vi "MasterAquisitionFile_FP_NoStim.vi"() -> ()   [LabVIEW 2020]
uses:
  <vilib>/vision/driver/IMAQdx.llb/IMAQdx Camera Control Mode.ctl
  <vilib>/vision/driver/IMAQdx.llb/IMAQdx Acquisition Mode.ctl
  <vilib>/userDefined/High Color/IMAQdx.ctl
  <vilib>/vision/driver/IMAQdx.llb/IMAQdx Buffer Number Mode.ctl
  <vilib>/DAQmx/read.llb/DAQmx Read (Digital 1D Bool 1Chan 1Samp).vi
  <vilib>/DAQmx/read.llb/DAQmx Read (Analog 1D Wfm NChan NSamp).vi
  <vilib>/DAQmx/create/channels.llb/DAQmx Create Channel (DI-Digital Input).vi
  <vilib>/DAQmx/miscellaneous.llb/DAQmx Fill In Error Info.vi
  <vilib>/DAQmx/create/channels.llb/DAQmx Create Channel (AI-Voltage-Basic).vi
  <vilib>/DAQmx/configure/timing.llb/DAQmx Timing (Sample Clock).vi
  <vilib>/DAQmx/configure/trigger.llb/DAQmx Start Trigger (Digital Edge).vi
  <vilib>/DAQmx/create/channels.llb/DAQmx Create Channel (CO-Pulse Generation-Frequency).vi
  <vilib>/DAQmx/configure/timing.llb/DAQmx Timing (Implicit).vi
  <vilib>/vision/driver/NI_Vision_Acquisition_Software.lvlib
  <resource>/objmgr/imaqdx.rc
panel:
  out "?":bool[](array[boolean])=[TRUE]
  out "Hexadecimal Data":u32=1 format="%x"
  out "Doric Trig":bool
  in  "Analog Input Channels":tag="Dev1/ai3:4, Dev1/ai7:13"
  out "?":T1(plugin-control)
  in  "stop":bool
  out "?":T1(plugin-control)
  out "Behavior Cam Fs":dbl(knob) scale=0.0..200.0
  out "Behav Cam":bool
  out "Whisk Cam":bool
  out "Analog Data":bool
  out "Time Elapsed (Min)":cluster{dbl, dbl}(slide)={16.0, 0.0} scale=0.0..16.0 scale format="%#_2g"
  out "Saving":bool
  out "Analog Samples":i32
  in  "Device Analog Channel Labels":string[](array[string])=["AudSol", "560LH", "forceSensor", "hipp", "cortRH", "cortLH", "EMG", "LPadSol", "RPadSol"]
  in  "?":cluster{"Analog Fs":u16}={"Analog Fs"=20000} {"Analog Fs" format="%0.0f"}
  in  "?":cluster{"WhiskerCam Fs":u16}={"WhiskerCam Fs"=150}
  out "Notes Size":i32=7
  out "Notes Reversed":string[](array[string])=["Experimenter", "Animal ID", "Isoflurane time", "Amplifier Gain", "Session ID", "Hemisphere", "Solenoid PSI"]
  out "Notes Array":string[](array[string])=["Solenoid PSI", "Hemisphere", "Session ID", "Amplifier Gain", "Isoflurane time", "Animal ID", "Experimenter"]
  in  "Notes:":T2={"Experimenter"="Kevin\n", "Animal ID"="T235", "Isoflurane time"="1250", "Amplifier Gain"="10000", "Session ID"="Imaging Session One", "Hemisphere"="RH", "Solenoid PSI"="10"}
  in  "Target Path":path=path "C:/Users/klt8/Documents/T236" caption="Final Saved File Location"
  out "Dropped":u32(slide) caption="WhiskerCam" scale=0.0..150.0
  out "Current File Name":string="210916_14_47_27"
  in  "Time (min)":dbl(knob)=15.5 min=0.5 max=20.0 step=0.5 scale=0.0..20.0 scale format="%#_3g"
  in  "Temp Path":path=path "C:/Users/klt8/Documents/LabVIEW Temp Data" caption="Temporary File Path"
  out "Last Whisk Buffer":u32
  out "Whisker Cam Fs":dbl(knob) scale=0.0..200.0 scale format="%#1_6g"
  # "Notes"
  # "Dropped Frames"
  # "Analog Fs"
  # "Whisker Fs"
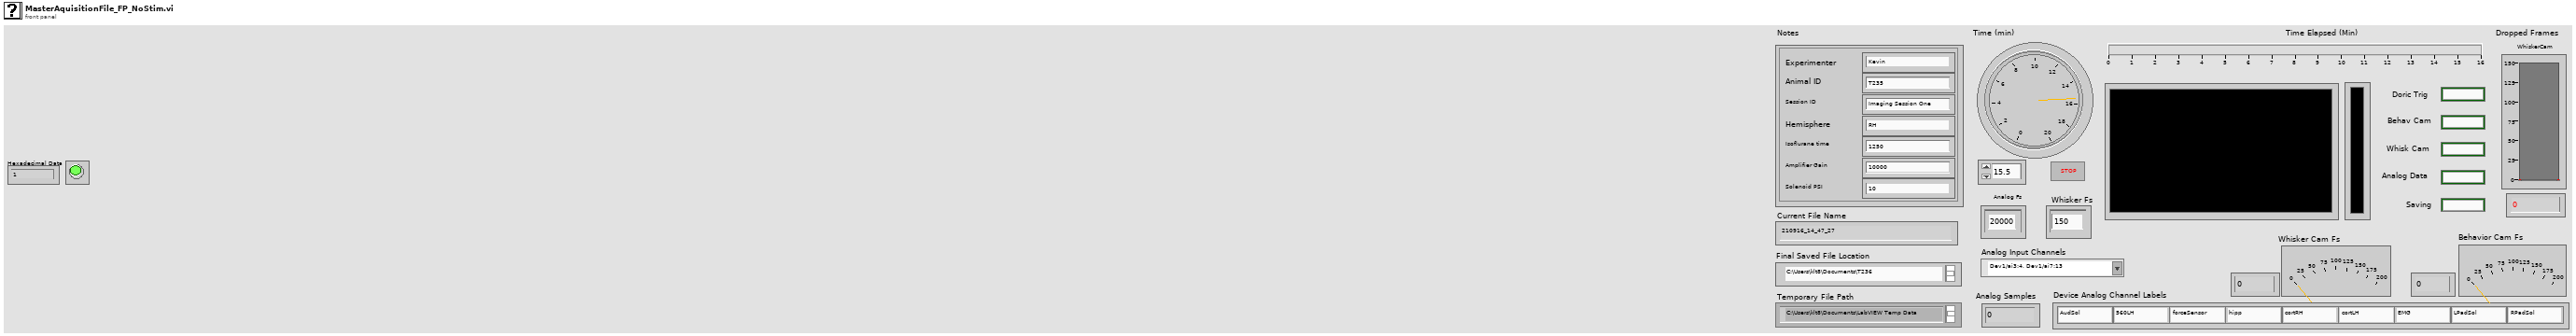
[diagram p1: front panel]
types:
  T1 = typedef "IMAQ Image.ctl" = refnum<image>
  T2 = cluster{"Experimenter":string, "Animal ID":string, "Isoflurane time":string, "Amplifier Gain":string, "Session ID":string, "Hemisphere":string, "Solenoid PSI":string}
  T3 = typedef "IMAQdx.ctl" = refnum<k21>
  T4 = enum16{"open", "open or create", "create or replace", "create", "open (read-only)"}
  T5 = typedef "NI_Vision_Acquisition_Software.lvlib/IMAQdx Camera Control Mode.ctl" = enum32{"Controller", "Listener"}
  T6 = enum16{"open", "replace", "create", "open or create", "replace or create", "replace or create with confirmation"}
  T7 = typedef "NI_Vision_Acquisition_Software.lvlib/IMAQdx Acquisition Mode.ctl" = enum32{"One Shot", "Continuous"}
  T8 = enum16{"big-endian, network order", "native, host order", "little-endian"}
  T9 = typedef "NI_Vision_Acquisition_Software.lvlib/IMAQdx Buffer Number Mode.ctl" = enum32{"Next", "Last", "Buffer Number", "Every", "Last New"}
  T10 = typedef "Image Type" = u32
  T11 = typedef "IMAQ AVI2 Refnum.ctl" = refnum<k20>
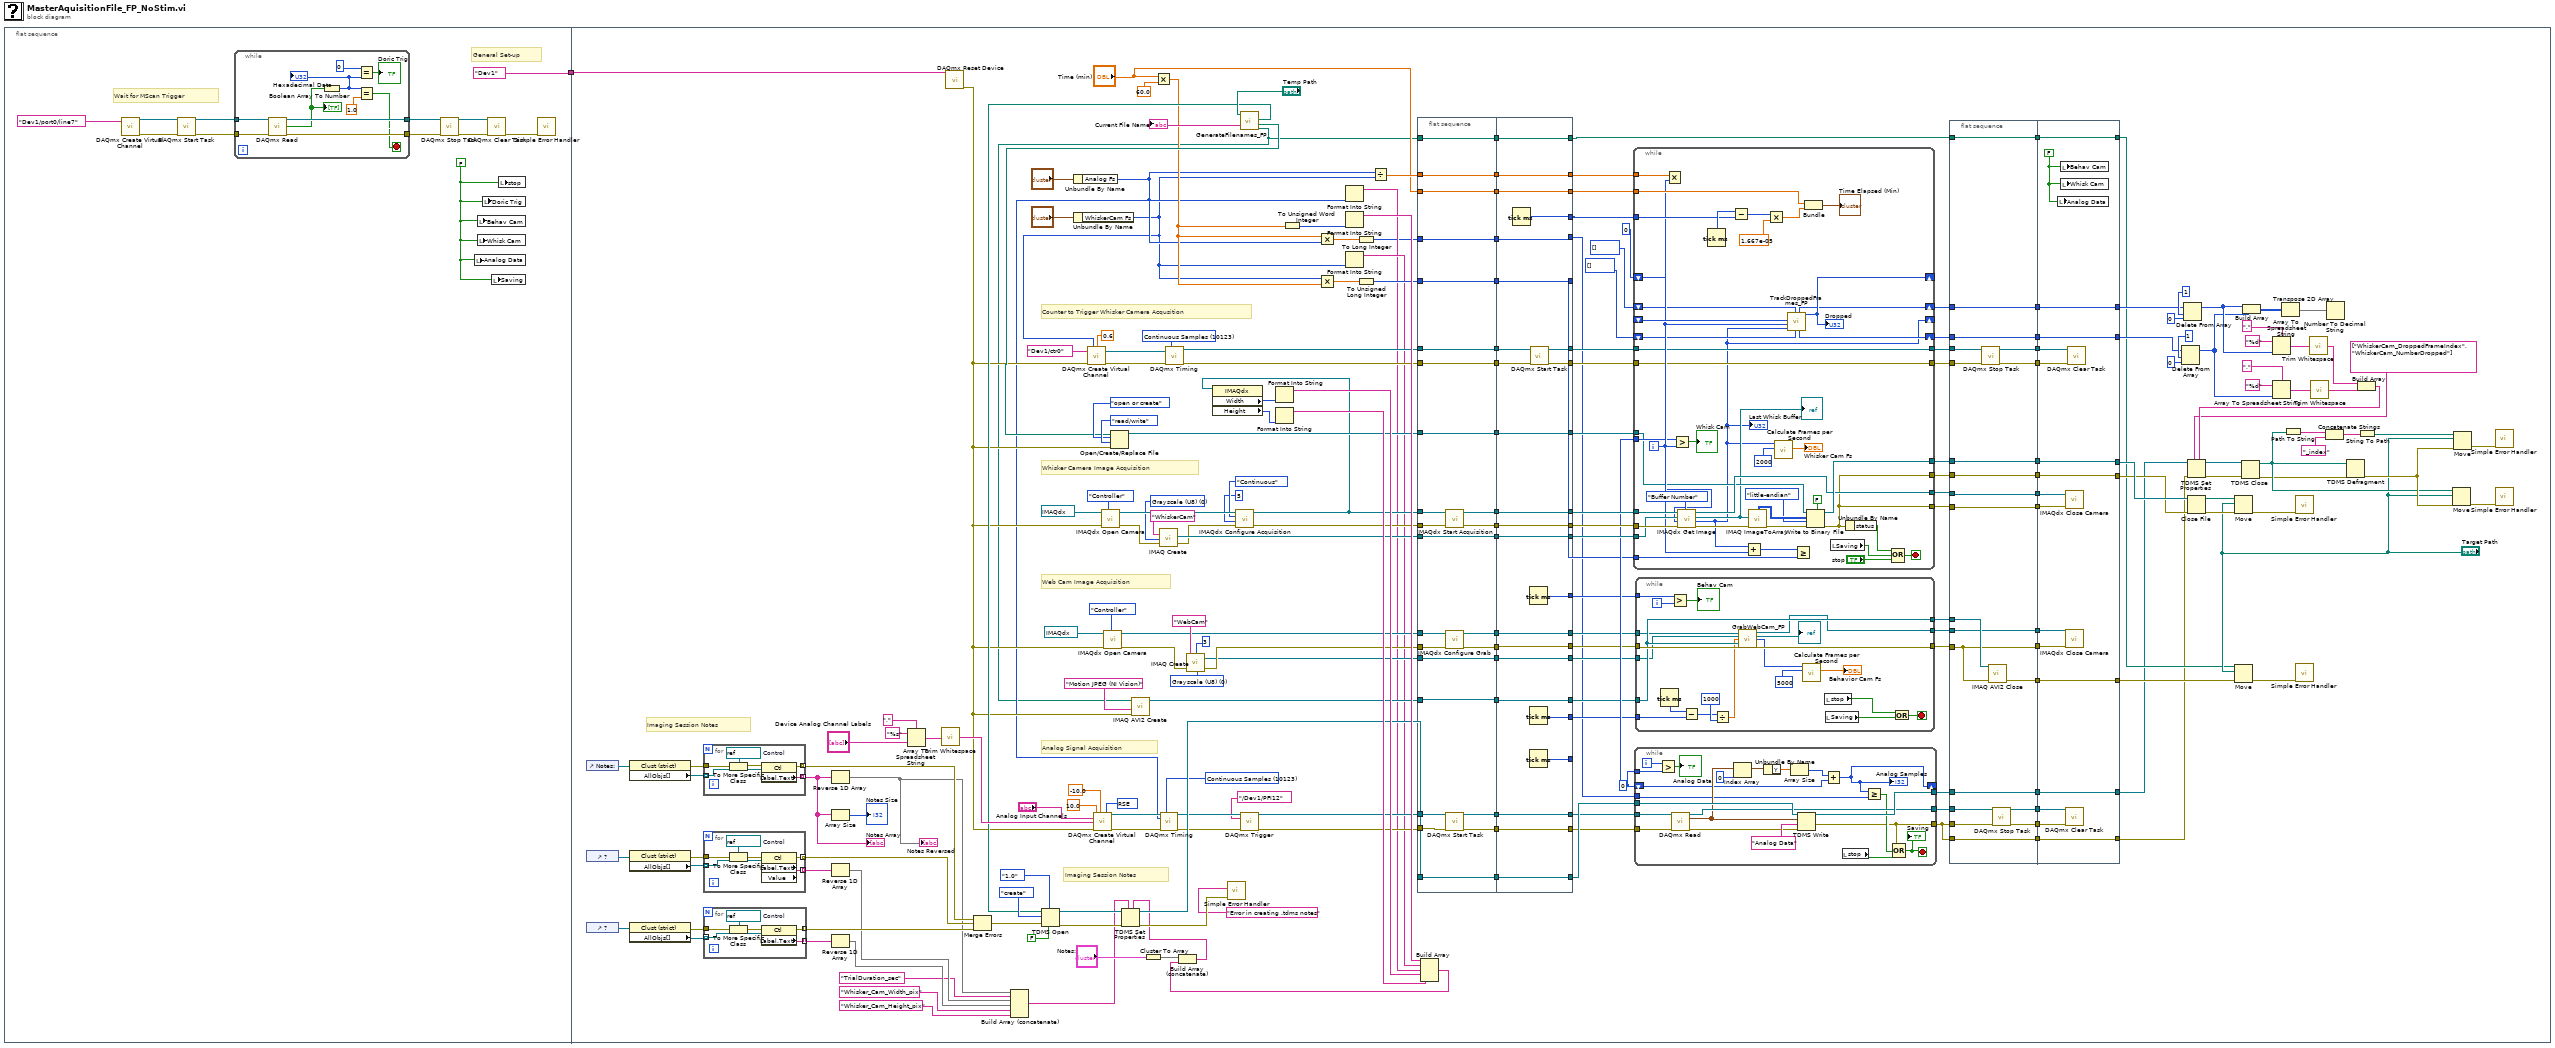
[diagram p0: block diagram]
diagram:
  n1 = flat-sequence {
    tunnel: [tag "Dev1" ("NI Board")] -> w1
    tunnel: w1 -> [w49]
    frame #0 {
      w2 = FALSE
      # "Wait for MScan Trigger"
      # "General Set-up"
      n2 = call-poly <vilib>:"DAQmx Create Virtual Channel.vi"("lines"=tag "Dev1/port0/line7" ("MScan Trigger")) -> ("task out"=w8:refnum<k21>, "error out"=w7:errorcluster)  [unwired: 13 in]
      n3 = call <vilib>:"DAQmx Start Task.vi"("task/channels in"=w8, "error in"=w7) -> ("task out"=w4:refnum<k21>, "error out"=w5:errorcluster)  [unwired: 12 in]
      n4 = while {
        tunnel: w4 -> [w23]
        tunnel: w5 -> [w22]
        tunnel: [w20] -> w10
        tunnel: [w21] -> w9
        stop <- w15 stop-if-true
        n5 = call-poly <vilib>:"DAQmx Read.vi"("task/channels in"=w23, "error in"=w22) -> ("task out"=w21:refnum<k21>, "data"=w19:bool[], "error out"=w20:errorcluster)  [unwired: 11 in]
        "?" <- w19
        n6 = Boolean Array To Number(Boolean array=w19) -> (number=w14:u32)
        "Hexadecimal Data" <- w14
        n7 = Equal?(x=w14, y=u32 0) -> (x = y?=→"Doric Trig":bool)
        n8 = Equal?(x=w14, y=1.0) -> (x = y?=w15:bool)
      }
      n9 = call <vilib>:"DAQmx Stop Task.vi"("task/channels in"=w9, "error in"=w10) -> ("task out"=w11:refnum<k21>, "error out"=w12:errorcluster)  [unwired: 12 in]
      n10 = local write "Analog Data"(w2) -> ()
      n11 = local write "Behav Cam"(w2) -> ()
      n12 = local write "Whisk Cam"(w2) -> ()
      n13 = local write "Doric Trig"(w2) -> ()
      n14 = call <vilib>:"DAQmx Clear Task.vi"("task in"=w11, "error in"=w12) -> ("error out"=w6:errorcluster)  [unwired: 13 in]
      n15 = local write "Saving"(w2) -> ()
      n16 = local write "stop"(w2) -> ()
      n17 = call <vilib>:"Simple Error Handler.vi"("error in (no error)"=w6) -> ()  [unwired: 4 in, 5 out]
    }
    frame #1 {
      w139 = T10 0 items=["Grayscale (U8)", "Grayscale (I16)", "Grayscale (SGL)", "Complex (CSG)", "RGB (U32)", "HSL (U32)", "RGB (U64)", "Grayscale (U16)"] ("Image Type")
      w131 = u32 0 ("y")
      w153 = 10123 items=["Finite Samples"=10178, "Continuous Samples"=10123, "Hardware Timed Single Point"=12522] ("sample mode")
      w152 = 10083 items=["default"=-1, "RSE"=10083, "NRSE"=10078, "Differential"=10106, "Pseudodifferential"=12529] ("input terminal configuration")
      w154 = 10123 items=["Finite Samples"=10178, "Continuous Samples"=10123, "Hardware Timed Single Point"=12522] ("sample mode")
      w150 = T10 0 items=["Grayscale (U8)", "Grayscale (I16)", "Grayscale (SGL)", "Complex (CSG)", "RGB (U32)", "HSL (U32)", "RGB (U64)", "Grayscale (U16)"] ("Image Type")
      # "Imaging Session Notes"
      # "Whisker Camera Image Acquisition"
      # "Imaging Session Notes"
      # "Counter to Trigger Whisker Camera Acqusition"
      # "Web Cam Image Acquisition"
      # "Analog Signal Acquisition"
      n18 = control-ref of="Notes:"() -> (w91:refnum<vi>)
      n19 = control-ref of="?"() -> (w93:refnum<vi>)
      n20 = control-ref of="?"() -> (w100:refnum<vi>)
      n21 = property class="Clust (strict)"(reference=w91) -> (error out=w92:errorcluster, "AllObjs[]"=w90:refnum<vi>[])  [unwired: 1 in, 1 out]
      n22 = property class="Clust (strict)"(reference=w93) -> (error out=w95:errorcluster, "AllObjs[]"=w94:refnum<vi>[])  [unwired: 1 in, 1 out]
      n23 = property class="Clust (strict)"(reference=w100) -> (error out=w99:errorcluster, "AllObjs[]"=w97:refnum<vi>[])  [unwired: 1 in, 1 out]
      n24 = for {
        tunnel: [w256] -> w85 mode=indexing
        tunnel: w90 -> [w255] mode=indexing
        tunnel: w92 -> [w254]
        tunnel: [w252] -> w86 mode=indexing
        w257 = refnum<vi> refnum  # Control
        n25 = To More Specific Class(target class=w257, reference=w255, error in=w254) -> (specific class reference=w258:refnum<vi>, error out=w253:errorcluster)
        n26 = property class="Ctl"(reference=w258, error in=w253) -> (error out=w252:errorcluster, "Label.Text"=w256:string)  [unwired: 1 out]
      }
      "Notes Array" <- w85
      n27 = for {
        tunnel: [w263] -> w96 mode=indexing
        tunnel: w94 -> [w262] mode=indexing
        tunnel: w95 -> [w261]
        tunnel: [w259] -> w87 mode=indexing
        w264 = refnum<vi> refnum  # Control
        n28 = To More Specific Class(target class=w264, reference=w262, error in=w261) -> (specific class reference=w265:refnum<vi>, error out=w260:errorcluster)
        n29 = property class="Ctl" props=["Label", "Text", "Value"](reference=w265, error in=w260) -> (error out=w259:errorcluster, "Label.Text"=w263:string)  [unwired: 2 out]
      }
      n30 = for {
        tunnel: [w270] -> w98 mode=indexing
        tunnel: w97 -> [w269] mode=indexing
        tunnel: w99 -> [w268]
        tunnel: [w266] -> w88 mode=indexing
        w271 = refnum<vi> refnum  # Control
        n31 = To More Specific Class(target class=w271, reference=w269, error in=w268) -> (specific class reference=w272:refnum<vi>, error out=w267:errorcluster)
        n32 = property class="Ctl"(reference=w272, error in=w267) -> (error out=w266:errorcluster, "Label.Text"=w270:string)  [unwired: 1 out]
      }
      n33 = Reverse 1D Array(array=w85) -> (reversed array=w84:string[])
      "Notes Reversed" <- w84
      n34 = Array Size(array=w85) -> (size(s)=→"Notes Size":i32)
      n35 = Reverse 1D Array(array=w96) -> (reversed array=w80:string[])
      n36 = Reverse 1D Array(array=w98) -> (reversed array=w79:string[])
      n37 = Array To Spreadsheet String(delimiter (Tab)=",", array="Device Analog Channel Labels", 3:"%s" ("format string")) -> (spreadsheet string=w83:string)
      n38 = call <vilib>:"Trim Whitespace.vi"("string"=w83) -> ("trimmed string"=w72:string)  [unwired: 1 in]
      n39 = call <vilib>:"DAQmx Reset Device.vi"("device in"=w49) -> ("error out"=w55:errorcluster)  [unwired: 14 in]
      n40 = Merge Errors(w86, w87, w88) -> (w71:errorcluster)
      n41 = Build Array (concatenate)(w84, "TrialDuration_sec", w80, w79, "Whisker_Cam_Width_pix", "Whisker_Cam_Height_pix") -> (w70:string[])
      n42 = Unbundle By Name("?") -> ("Analog Fs"=w53:u16)
      n43 = Unbundle By Name("?") -> ("WhiskerCam Fs"=w52:u16)
      n44 = call-poly <vilib>:"DAQmx Create Virtual Channel.vi"("frequency"=w52, "duty cycle"=0.6, "counter"=tag "Dev1/ctr0" ("Whisk Cam Counter"), "error in"=w55) -> ("task out"=w177:refnum<k21>, "error out"=w178:errorcluster)  [unwired: 10 in]
      n45 = call-poly <vilib>:"DAQmx Create Virtual Channel.vi"("maximum value"=10.0, "minimum value"=-10.0, "input terminal configuration"=w152, "physical channels"="Analog Input Channels", "name to assign"=w72, "error in"=w55) -> ("task out"=w185:refnum<k21>, "error out"=w186:errorcluster)  [unwired: 8 in]
      n46 = call <vilib>:"IMAQdx Open Camera.vi"("Camera Control Mode"=IMAQdx_Camera_Control_Mode."Controller", "error in"=w55, "Session In"=T3 "cam1" ("Whisker Cam ID")) -> ("error out"=w175:errorcluster, "Session Out"=w174:T3)  [unwired: 7 in]
      n47 = call <vilib>:"IMAQdx Open Camera.vi"("Camera Control Mode"=IMAQdx_Camera_Control_Mode."Controller", "error in"=w55, "Session In"=T3 "cam0" ("WebCam ID")) -> ("error out"=w136:errorcluster, "Session Out"=w135:T3)  [unwired: 7 in]
      n48 = Cluster To Array(cluster="Notes:") -> (array=w73:string[])
      n49 = Multiply(x="Time (min)", y=60.0) -> (x*y=w54:dbl)
      n50 = call "IMAQ Create"("Image Name"="WhiskerCam", "Image Type"=w150, "error in (no error)"=w175) -> ("New Image"=w210:T1, "error out"=w176:errorcluster)  [unwired: 2 in]
      n51 = call-poly <vilib>:"DAQmx Timing.vi"("task/channels in"=w185, "sample mode"=w153, "rate"=w53, "error in"=w186) -> ("task out"=w187:refnum<k21>, "error out"=w188:errorcluster)  [unwired: 10 in]
      n52 = call-poly <vilib>:"DAQmx Timing.vi"("task/channels in"=w177, "sample mode"=w154, "error in"=w178) -> ("task out"=w194:refnum<k21>, "error out"=w195:errorcluster)  [unwired: 11 in]
      n53 = call "IMAQ Create"("Border Size"=3, "Image Name"="WebCam", "Image Type"=w139, "error in (no error)"=w136) -> ("New Image"=w133:T1, "error out"=w134:errorcluster)  [unwired: 1 in]
      n54 = call <vilib>:"IMAQdx Configure Acquisition.vi"("error in"=w176, "Number of Buffers"=u32 5, "Continuous?"=IMAQdx_Acquisition_Mode."Continuous", "Session In"=w174) -> ("error out"=w179:errorcluster, "Session Out"=w119:T3)  [unwired: 6 in]
      n55 = property class="IMAQdx"(reference=w119) -> ("Width"=w208:u32, "Height"=w209:u32)  [unwired: 1 in, 2 out]
      n56 = call "GenerateFilenames_FP.vi"("path"="Temp Path") -> ("WebCam Path"=w34:path, "Basler Path"=w60:path, "TDMS Path"=w59:path, "Analog file name"=→"Current File Name":string)  [unwired: 2 in, 1 out]
      n57 = TDMS Open(6:FALSE ("disable buffering? (T)"), 7:enum16{"1.0", "2.0"}."1.0" ("file format version (2.0)"), 8:w71, 10:T4."create" ("operation (0:open)"), 11:w59) -> (0:w121:errorcluster, 3:w120:refnum<k34>)  [unwired: 2 in]
      n58 = Open/Create/Replace File(file path (use dialog)=w60, error in=w55, operation (0:open)=T6."open or create", access (0:read/write)=enum16{"read/write", "read-only", "write-only"}."read/write") -> (refnum out=w184:refnum<file>)  [unwired: 2 in, 2 out]
      n59 = call "IMAQ AVI2 Create"("error in (no error)"=w55, "Codec"="Motion JPEG (NI Vision)", "AVI Path"=w34) -> ("AVI Refnum"=w127:T11)  [unwired: 7 in, 1 out]
      n60 = call-poly <vilib>:"DAQmx Trigger.vi"("task/channels in"=w187, "source"=tag "/Dev1/PFI12" ("Whisk Cam Trigger"), "error in"=w188) -> ("task out"=w189:refnum<k21>, "error out"=w190:errorcluster)  [unwired: 11 in]
      n61 = Format Into String(w208) -> (resulting string=w224:string)  [unwired: 3 in, 1 out]
      n62 = Format Into String(w209) -> (resulting string=w223:string)  [unwired: 3 in, 1 out]
      n63 = To Unsigned Word Integer(number=w54) -> (unsigned 16bit integer=w207:u16)
      n64 = Multiply(x=w54, y=w53) -> (x*y=w36:dbl)
      n65 = Multiply(x=w52, y=w54) -> (x*y=w217:dbl)
      n66 = Format Into String(w53) -> (resulting string=w56:string)  [unwired: 3 in, 1 out]
      n67 = Format Into String(w207) -> (resulting string=w225:string)  [unwired: 3 in, 1 out]
      n68 = Format Into String(w52) -> (resulting string=w57:string)  [unwired: 3 in, 1 out]
      n69 = To Long Integer(number=w36) -> (32bit integer=w35:i32)
      n70 = To Unsigned Long Integer(number=w217) -> (unsigned 32bit integer=w218:u32)
      n71 = Divide ("An_Fs/Whisk_Fs ratio")(x=w53, y=w52) -> (x/y=w61:dbl)
      n72 = flat-sequence {
        tunnel: w119 -> [w377]
        tunnel: w179 -> [w376]
        tunnel: [w375] -> w251
        tunnel: [w374] -> w250
        tunnel: [w373] -> w249
        tunnel: w210 -> [w373]
        tunnel: [w372] -> w248
        tunnel: w184 -> [w372]
        tunnel: w189 -> [w371]
        tunnel: w190 -> [w370]
        tunnel: [w369] -> w247
        tunnel: [w368] -> w246
        tunnel: [w367] -> w245
        tunnel: w205 -> [w367]
        tunnel: w194 -> [w366]
        tunnel: [w366] -> w244
        tunnel: w195 -> [w365]
        tunnel: [w365] -> w243
        tunnel: w35 -> [w364]
        tunnel: [w364] -> w242
        tunnel: w218 -> [w363]
        tunnel: [w363] -> w241
        tunnel: "Time (min)" -> [w362]
        tunnel: [w362] -> w240
        tunnel: w135 -> [w361]
        tunnel: w134 -> [w360]
        tunnel: w133 -> [w359]
        tunnel: [w359] -> w239
        tunnel: [w358] -> w238
        tunnel: [w357] -> w237
        tunnel: [w356] -> w236
        tunnel: w127 -> [w356]
        tunnel: [w355] -> w235
        tunnel: w61 -> [w355]
        tunnel: w34 -> [w354]
        tunnel: [w354] -> w33
        tunnel: [w394] -> w143
        tunnel: [w393] -> w144
        tunnel: [w401] -> w180
        tunnel: w251 -> [w401]
        tunnel: [w400] -> w181
        tunnel: w250 -> [w400]
        tunnel: [w399] -> w182
        tunnel: w249 -> [w399]
        tunnel: [w398] -> w183
        tunnel: w248 -> [w398]
        tunnel: [w397] -> w192
        tunnel: w247 -> [w397]
        tunnel: [w396] -> w191
        tunnel: w246 -> [w396]
        tunnel: [w395] -> w193
        tunnel: w245 -> [w395]
        tunnel: w244 -> [w390]
        tunnel: w243 -> [w392]
        tunnel: w242 -> [w379]
        tunnel: w241 -> [w391]
        tunnel: [w391] -> w116
        tunnel: [w389] -> w173
        tunnel: w240 -> [w388]
        tunnel: [w388] -> w142
        tunnel: [w387] -> w130
        tunnel: w239 -> [w387]
        tunnel: [w386] -> w128
        tunnel: w238 -> [w386]
        tunnel: [w385] -> w129
        tunnel: w237 -> [w385]
        tunnel: [w384] -> w125
        tunnel: w236 -> [w383]
        tunnel: [w383] -> w126
        tunnel: [w382] -> w124
        tunnel: [w379] -> w115
        tunnel: [w381] -> _
        tunnel: [w380] -> w110
        tunnel: w235 -> [w380]
        tunnel: [w378] -> w31
        tunnel: w33 -> [w378]
        frame #0 {
          n73 = call <vilib>:"IMAQdx Start Acquisition.vi"("error in"=w376, "Session In"=w377) -> ("error out"=w374:errorcluster, "Session Out"=w375:T3)  [unwired: 8 in]
          n74 = call <vilib>:"IMAQdx Configure Grab.vi"("error in"=w360, "Session In"=w361) -> ("error out"=w357:errorcluster, "Session Out"=w358:T3)  [unwired: 8 in]
          n75 = call <vilib>:"DAQmx Start Task.vi"("task/channels in"=w371, "error in"=w370) -> ("task out"=w369:refnum<k21>, "error out"=w368:errorcluster)  [unwired: 12 in]
        }
        frame #1 {
          n76 = Tick Count (ms)() -> (millisecond timer value=w389:u32)
          n77 = Tick Count (ms)() -> (millisecond timer value=w384:u32)
          n78 = Tick Count (ms)() -> (millisecond timer value=w382:u32)
          n79 = Tick Count (ms)() -> (millisecond timer value=w381:u32)
          n80 = call <vilib>:"DAQmx Start Task.vi"("task/channels in"=w390, "error in"=w392) -> ("task out"=w394:refnum<k21>, "error out"=w393:errorcluster)  [unwired: 12 in]
        }
      }
      n81 = Build Array(w225, w57, w56, w224, w223) -> (w117:string[])
      n82 = Build Array (concatenate)(w73, w117) -> (w145:string[])
      n83 = TDMS Set Properties(5:w145, 7:w70, 8:w121, 11:w120) -> (0:w206:errorcluster, 3:w205:refnum<k34>)  [unwired: 2 in, 2 out]
      n84 = call <vilib>:"Simple Error Handler.vi"("error source (\" \")"="Error in creating .tdms notes" ("error source (\" \")"), "error in (no error)"=w206) -> ()  [unwired: 3 in, 5 out]
      n85 = while {
        tunnel: [w429] -> w101
        tunnel: [w415] -> w38
        tunnel: [w437] -> w41
        tunnel: w180 -> [w436]
        tunnel: w181 -> [w435]
        tunnel: w182 -> [w434]
        tunnel: w183 -> [w409]
        shift-right: [w406] -> _
        shift-left: _ -> [w433]
        shift-right: [w432] -> _
        shift-left: u32 0 ("New Lost") -> [w428]
        shift-right: [w431] -> w47
        shift-left: u32[] [] ("NewBuffNum") -> [w405]
        shift-right: [w430] -> w43
        shift-left: u32[] [] ("NewNumLost") -> [w424]
        tunnel: w116 -> [w426]
        tunnel: w173 -> [w419]
        tunnel: w142 -> [w417]
        tunnel: [w415] -> w102
        tunnel: w131 -> [w414]
        tunnel: w144 -> [w412]
        tunnel: w143 -> [w411]
        tunnel: [w412] -> w108
        tunnel: [w411] -> w109
        tunnel: w110 -> [w407]
        i -> [w404]
        stop <- w425 stop-if-true
        n86 = Multiply(x=w407, y=w404) -> ()  [unwired: 1 out]
        n87 = Greater?(x=w404, y=w414) -> (0:→"Whisk Cam":bool)
        n88 = call <vilib>:"IMAQdx Get Image.vi"("Buffer Number Mode (Next)"=IMAQdx_Buffer_Number_Mode."Buffer Number", "error in"=w435, "Buffer Number In"=w404, "Image In"=w434, "Session In"=w436) -> ("error out"=w443:errorcluster, "Buffer Number Out"=w406:u32, "Image Out"=w408:T1, "Session Out"=w429:T3)  [unwired: 3 in]
        "Last Whisk Buffer" <- w406
        "?" <- w408
        n89 = Tick Count (ms)() -> (millisecond timer value=w420:u32)
        n90 = Subtract(x=w420, y=w419) -> (x-y=w423:u32)
        n91 = Add(x=w406, y=w428) -> (x+y=w427:u32)
        n92 = call "IMAQ ImageToArray"("error in (no error)"=w443, "Image"=w408) -> ("error out"=w442:errorcluster, "Image Pixels (U8)"=w441:u8[][])  [unwired: 2 in, 3 out]
        n93 = Multiply(x=w423, y=1.667e-05) -> (x*y=w422:dbl)
        n94 = call <vilib>:"Calculate Frames per Second.vi"("Update Interval (ms)"=u32 2000, "Buffer Number"=w406) -> ("Processed Frames/s"=→"Whisker Cam Fs":dbl)  [unwired: 7 in, 2 out]
        n95 = call "TrackDroppedFrames_FP.vi"("NumLost"=w424, "BuffNum"=w405, "Curr Buffer"=w406, "Prev Lost"=w428, "Prev Buffer"=w433) -> ("New Lost"=w432:u32, "NewNumLost"=w430:u32[], "NewBuffNum"=w431:u32[])  [unwired: 4 in]
        "Dropped" <- w432
        n96 = Greater Or Equal?(x=w427, y=w426) -> ()  [unwired: 1 out]
        n97 = Bundle("Time (min)"=w417, w422) -> (→"Time Elapsed (Min)":cluster{"Time (min)":dbl, dbl})  [unwired: 1 in]
        n98 = Write to Binary File(file (use dialog)=w409, data=w441, error in=w442, 5:FALSE ("prepend array or string size? (T)"), 9:T8."little-endian" ("byte order (0:big-endian, network order)")) -> (refnum out=w437:refnum<file>, error out=w415:errorcluster)  [unwired: 1 in, 1 out]
        n99 = local read "Saving"() -> (w402:bool)
        n100 = Unbundle By Name(w415) -> ("status"=w403:bool)
        n101 = Compound Arithmetic op=OR(w403, w402, "stop") -> (w425:bool)
      }
      n102 = while {
        tunnel: w191 -> [w353]
        tunnel: w192 -> [w352]
        tunnel: w193 -> [w351]
        tunnel: [w350] -> w28
        tunnel: [w338] -> w26
        tunnel: [w349] -> w107
        shift-right: [w342] -> _
        shift-left: w131 -> [w343]
        tunnel: w131 -> [w334]
        tunnel: w115 -> [w332]
        i -> [w335]
        stop <- w339 stop-if-true
        n103 = Greater?(x=w335, y=w334) -> (0:→"Analog Data":bool)
        n104 = call-poly <vilib>:"DAQmx Read.vi"("task/channels in"=w352, "error in"=w353) -> ("task out"=w349:refnum<k21>, "data"=w347:waveform(dbl)[], "error out"=w341:errorcluster)  [unwired: 11 in]
        n105 = Index Array(array=w347, index=0) -> (element=w345:waveform(dbl))
        n106 = Unbundle By Name(w345) -> ("Y"=w344:dbl[])
        n107 = Array Size(array=w344) -> (size(s)=w337:i32)
        n108 = TDMS Write(0:w351, 5:"Analog Data" ("group name in (Untitled)"), 9:w347, 11:w341) -> (4:w350:refnum<k34>, 15:w338:errorcluster)  [unwired: 2 in, 2 out]
        n109 = Add(x=w337, y=w343) -> (x+y=w342:u32)
        "Analog Samples" <- w342
        n110 = local read "stop"() -> (w333:bool)
        n111 = Greater Or Equal?(x=w342, y=w332) -> (x >= y?=w340:bool)
        n112 = Compound Arithmetic op=OR(w333, w338, w340) -> (w339:bool)
        "Saving" <- w339
      }
      n113 = while {
        tunnel: w130 -> [w318]
        tunnel: w128 -> [w317]
        tunnel: w129 -> [w321]
        tunnel: w126 -> [w320]
        tunnel: [w311] -> w103
        tunnel: [w322] -> w104
        tunnel: [w320] -> w106
        tunnel: w125 -> [w324]
        tunnel: w124 -> [w323]
        i -> [w325]
        stop <- w313 stop-if-true
        n114 = Tick Count (ms)() -> (millisecond timer value=w329:u32)
        n115 = Greater?(x=w324, y=w325) -> (0:→"Behav Cam":bool)
        n116 = Subtract(x=w329, y=w323) -> (x-y=w330:u32)
        n117 = Divide(x=w330, y=u32 1000) -> (x/y=w319:dbl)
        n118 = call "GrabWebCam_FP.vi"("Session In"=w317, "Image In"=w318, "Trial Time"=w319, "AVI Refnum"=w320, "error in"=w321) -> ("Session Out"=w311:T3, "WebCam Img Out"=→"?":T1, "Buffer Number Out"=w315:u32, "error out"=w322:errorcluster)  [unwired: 7 in]
        n119 = call <vilib>:"Calculate Frames per Second.vi"("Update Interval (ms)"=u32 5000, "Buffer Number"=w315) -> ("Processed Frames/s"=→"Behavior Cam Fs":dbl)  [unwired: 7 in, 2 out]
        n120 = local read "stop"() -> (w312:bool)
        n121 = local read "Saving"() -> (w314:bool)
        n122 = Compound Arithmetic op=OR(w312, w314) -> (w313:bool)
      }
      n123 = flat-sequence {
        tunnel: w109 -> [w293]
        tunnel: w108 -> [w292]
        tunnel: [w291] -> w234
        tunnel: [w290] -> w233
        tunnel: [w289] -> w232
        tunnel: [w288] -> w231
        tunnel: w107 -> [w287]
        tunnel: w26 -> [w286]
        tunnel: w104 -> [w282]
        tunnel: w106 -> [w285]
        tunnel: [w284] -> w230
        tunnel: [w283] -> w229
        tunnel: w103 -> [w283]
        tunnel: [w282] -> w228
        tunnel: w102 -> [w281]
        tunnel: [w281] -> w227
        tunnel: w101 -> [w280]
        tunnel: [w280] -> w226
        tunnel: w47 -> [w279]
        tunnel: [w279] -> w46
        tunnel: [w278] -> w44
        tunnel: w43 -> [w278]
        tunnel: [w277] -> w42
        tunnel: w41 -> [w277]
        tunnel: [w276] -> w39
        tunnel: w38 -> [w276]
        tunnel: [w275] -> w32
        tunnel: w31 -> [w275]
        tunnel: w28 -> [w274]
        tunnel: [w274] -> w27
        tunnel: w26 -> [w273]
        tunnel: [w273] -> w25
        tunnel: w234 -> [w310]
        tunnel: w233 -> [w309]
        tunnel: w232 -> [w308]
        tunnel: w231 -> [w307]
        tunnel: w230 -> [w306]
        tunnel: [w306] -> w105
        tunnel: w229 -> [w305]
        tunnel: w228 -> [w304]
        tunnel: w227 -> [w303]
        tunnel: w226 -> [w302]
        tunnel: [w300] -> w48
        tunnel: w46 -> [w300]
        tunnel: [w299] -> w45
        tunnel: w44 -> [w299]
        tunnel: [w298] -> w40
        tunnel: w42 -> [w298]
        tunnel: w39 -> [w297]
        tunnel: [w297] -> w37
        tunnel: w32 -> [w296]
        tunnel: [w296] -> w30
        tunnel: [w295] -> w29
        tunnel: w27 -> [w295]
        tunnel: [w294] -> w24
        tunnel: w25 -> [w294]
        frame #0 {
          n124 = call <vilib>:"DAQmx Stop Task.vi"("task/channels in"=w293, "error in"=w292) -> ("task out"=w290:refnum<k21>, "error out"=w291:errorcluster)  [unwired: 12 in]
          n125 = call "IMAQ AVI2 Close"("error in (no error)"=w282, "AVI Refnum"=w285) -> ("error out"=w284:errorcluster)  [unwired: 9 in]
          n126 = call <vilib>:"DAQmx Stop Task.vi"("task/channels in"=w287, "error in"=w286) -> ("task out"=w289:refnum<k21>, "error out"=w288:errorcluster)  [unwired: 12 in]
        }
        frame #1 {
          w301 = FALSE
          n127 = local write "Analog Data"(w301) -> ()
          n128 = local write "Behav Cam"(w301) -> ()
          n129 = local write "Whisk Cam"(w301) -> ()
          n130 = call <vilib>:"IMAQdx Close Camera.vi"("error in"=w303, "Session In"=w302) -> ()  [unwired: 9 in, 1 out]
          n131 = call <vilib>:"IMAQdx Close Camera.vi"("error in"=w304, "Session In"=w305) -> ()  [unwired: 9 in, 1 out]
          n132 = call <vilib>:"DAQmx Clear Task.vi"("task in"=w308, "error in"=w307) -> ()  [unwired: 13 in, 1 out]
          n133 = call <vilib>:"DAQmx Clear Task.vi"("task in"=w309, "error in"=w310) -> ()  [unwired: 13 in, 1 out]
        }
      }
      n134 = Delete From Array(array=w45, length=1, index=0) -> (array with subset deleted=w221:u32[])  [unwired: 1 out]
      n135 = Delete From Array(array=w48, length=1, index=0) -> (array with subset deleted=w222:u32[])  [unwired: 1 out]
      n136 = Close File(refnum=w40, error in=w37) -> (path=w197:path, error out=w198:errorcluster)
      n137 = Move(source path=w197, error in=w198, 10:"Target Path") -> (error out=w200:errorcluster)  [unwired: 2 in, 2 out]
      n138 = Move(source path=w30, error in=w105, 10:"Target Path") -> (error out=w132:errorcluster)  [unwired: 2 in, 2 out]
      n139 = Build Array(w222, w221) -> (w219:u32[][])
      n140 = Array To Spreadsheet String(delimiter (Tab)=",", array=w222, 3:"%d" ("format string")) -> (spreadsheet string=w213:string)
      n141 = Array To Spreadsheet String(delimiter (Tab)=",", array=w221, 3:"%d" ("format string")) -> (spreadsheet string=w214:string)
      n142 = Transpose 2D Array(2D array=w219) -> (transposed array=w220:u32[][])
      n143 = call <vilib>:"Simple Error Handler.vi"("error in (no error)"=w200) -> ()  [unwired: 1 in, 8 out]
      n144 = call <vilib>:"Simple Error Handler.vi"("error in (no error)"=w132) -> ()  [unwired: 1 in, 8 out]
      n145 = call <vilib>:"Trim Whitespace.vi"("string"=w213) -> ("trimmed string"=w114:string)  [unwired: 1 in]
      n146 = call <vilib>:"Trim Whitespace.vi"("string"=w214) -> ("trimmed string"=w215:string)  [unwired: 1 in]
      n147 = Number To Decimal String(number=w220) -> ()  [unwired: 1 in, 1 out]
      n148 = Build Array(w114, w215) -> (w216:string[])
      n149 = TDMS Set Properties(5:w216, 7:string[] ["WhiskerCam_DroppedFrameIndex", "WhiskerCam_NumberDropped"] ("channel name(s) in (Untitled)"), 8:w24, 11:w29) -> (0:w211:errorcluster, 3:w212:refnum<k34>)  [unwired: 2 in, 2 out]
      n150 = TDMS Close(8:w211, 11:w212) -> (0:w196:errorcluster, 3:w201:path)
      n151 = Path To String(path=w201) -> (string=w113:string)
      n152 = Concatenate Strings(w113, "_index" ("string")) -> (w202:string)
      n153 = TDMS Defragment(4:w196, 7:w201) -> (0:w204:errorcluster)
      n154 = String To Path(string=w202) -> (path=w203:path)
      n155 = Move(source path=w201, error in=w204, 10:"Target Path") -> (error out=w199:errorcluster)  [unwired: 2 in, 2 out]
      n156 = Move(source path=w203, error in=w204, 10:"Target Path") -> (error out=w112:errorcluster)  [unwired: 2 in, 2 out]
      n157 = call <vilib>:"Simple Error Handler.vi"("error in (no error)"=w112) -> ()  [unwired: 1 in, 8 out]
      n158 = call <vilib>:"Simple Error Handler.vi"("error in (no error)"=w199) -> ()  [unwired: 1 in, 8 out]
    }
  }
